vi "FCPConnect.vi"(11 "FPGA IP Address":string) -> (0 "error out":errorcluster, 1 "Sequence Number":i32, 2 "FPGA IP Address Out":u32, 3 "connection ID out":refnum<k16>)   [LabVIEW 2009]
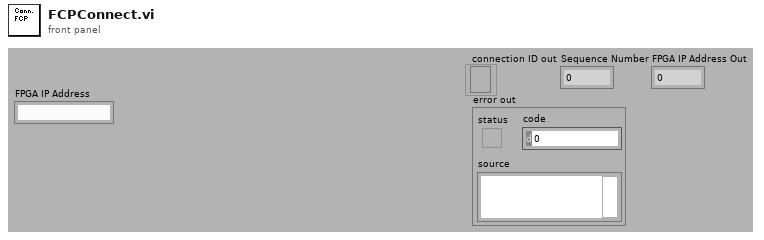
[diagram p1: front panel]
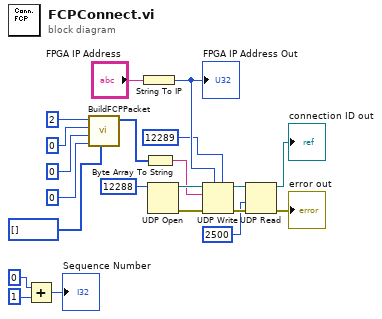
[diagram p0: block diagram]
diagram:
  n1 = Add(x=0, y=1) -> (x+y=→"Sequence Number":i32)
  n2 = call "BuildFCPPacket.vi"("Data"=u32[] [], "Data Length (in Bytes)"=u32 0, "SequenceNumber"=u32 0, "Channel"=u32 0, "Command"=u32 2) -> ("FCP Packet"=w6:u32[])  [unwired: 6 in]
  n3 = String To IP(1:"FPGA IP Address") -> (0:w19:u32)
  "FPGA IP Address Out" <- w19
  n4 = Byte Array To String(unsigned byte array=w6) -> (string=w16:string)
  n5 = UDP Open(11:u16 12288 ("port")) -> (port=w21:refnum<k16>, 0:w20:errorcluster)  [unwired: 4 in, 1 out]
  n6 = UDP Write(address=w19, port or service name=u16 12289, connection ID=w21, data in=w16, 8:w20) -> (error out=w14:errorcluster, 3:w15:refnum<k16>)  [unwired: 1 in]
  n7 = UDP Read(connection ID=w15, timeout ms (25000)=2500, 8:w14) -> (error out=→"error out":errorcluster, 3:→"connection ID out":refnum<k16>)  [unwired: 1 in, 3 out]
